vi "SSI_Trig In Array.vi"(1 "Trig_Count":u8[](array[numeric]), 2 "Input Array":dbl[][](array[numeric]), 3 "Group":i32) -> (0 "Output Array":dbl[][](array[numeric]))   [LabVIEW 2011]
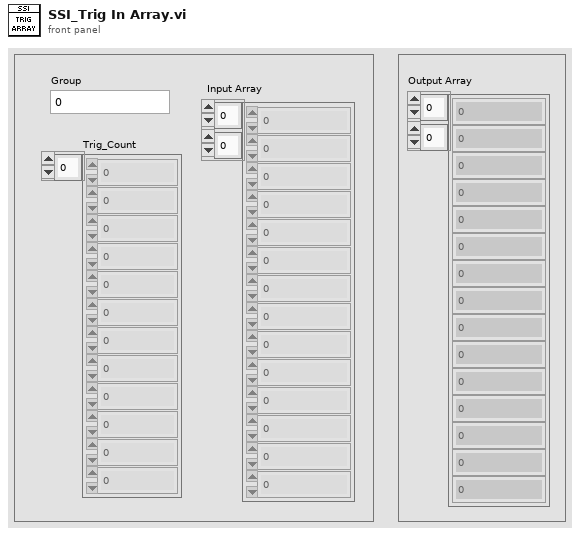
[diagram p1: front panel]
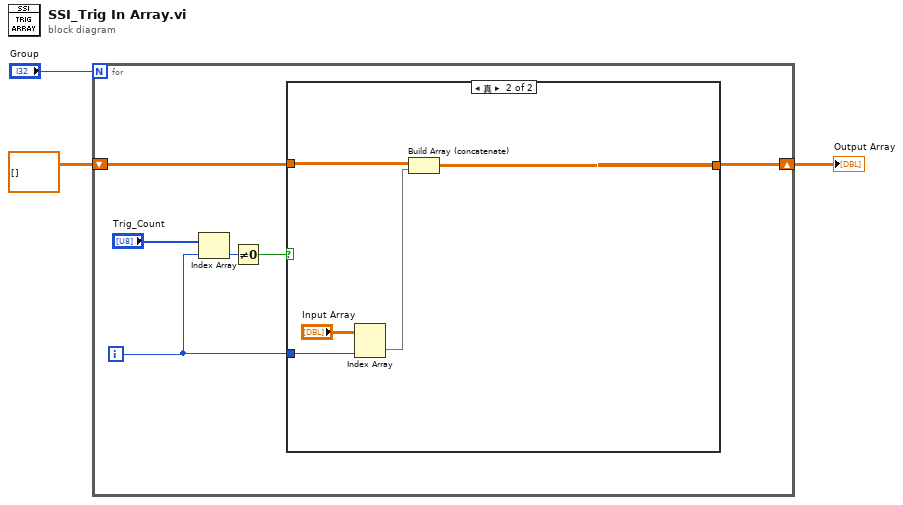
[diagram p0: block diagram]
diagram:
  n1 = for {
    N: "Group" -> [_]
    shift-right: [w7] -> w1
    shift-left: dbl[][] [] -> [w9]
    i -> [w8]
    n2 = Index Array(array="Trig_Count", index=w8) -> (element=w5:u8)
    n3 = Not Equal To 0?(x=w5) -> (x != 0?=w6:bool)
    n4 = case shown="真" w6 {
      tunnel: w9 -> [w10 w15]
      tunnel: [w10 w11] -> w7
      tunnel: w8 -> [_ w14]
      frame False {
      }
      frame True {
        n5 = Index Array(array="Input Array", index (col)=w14) -> (element=w12:dbl[])  [unwired: 1 in]
        n6 = Build Array (concatenate)(w15, w12) -> (w11:dbl[][])
      }
    }
  }
  "Output Array" <- w1
